vi "Render List.vi"(10 "Value":i32, 11 "Display State In":T2={"Persistent"={"Elements"=[], "PicElements"=[], "Limits"=[], "Selection"=[], "Selection Color"=0, "Highlight"=[], "Highlight Val"=0, "Highlight Color"={"Back"=0, "Edge"=0}, "Font"={"Details"={"Font Name:"="Lucida Sans", "Size"=24, "Strikeout?"=FALSE, "Italic?"=FALSE, "Underline?"=FALSE, "Outline?"=FALSE, "Shadow?"=FALSE, "Bold?"=TRUE}, "Color"=7697781}, "Bakground Color"=0}, "List Ref"=refnum, "nbVisible"=0, "FirstIdx"=0, "More.Width"=0} caption="State") -> (0 "OutOfBounds":bool, 2 "Selection":picture, 3 "Display State Out":T2={"Persistent"={"Elements"=[], "PicElements"=[], "Limits"=[], "Selection"=[], "Selection Color"=0, "Highlight"=[], "Highlight Val"=0, "Highlight Color"={"Back"=0, "Edge"=0}, "Font"={"Details"={"Font Name:"="Lucida Sans", "Size"=24, "Strikeout?"=FALSE, "Italic?"=FALSE, "Underline?"=FALSE, "Outline?"=FALSE, "Shadow?"=FALSE, "Bold?"=TRUE}, "Color"=7697781}, "Bakground Color"=0}, "List Ref"=refnum, "nbVisible"=0, "FirstIdx"=0, "More.Width"=0} caption="State", 5 "Actual Value":T1 caption="s? t:f")   [LabVIEW 2016, in "Horizontal MenuList.xctl"]
uses:
  Horizontal MenuList.xctl
  Horizontal MenuList_State.ctl
  Highlight Colors.ctl
  Horizontal MenuList_Data.ctl
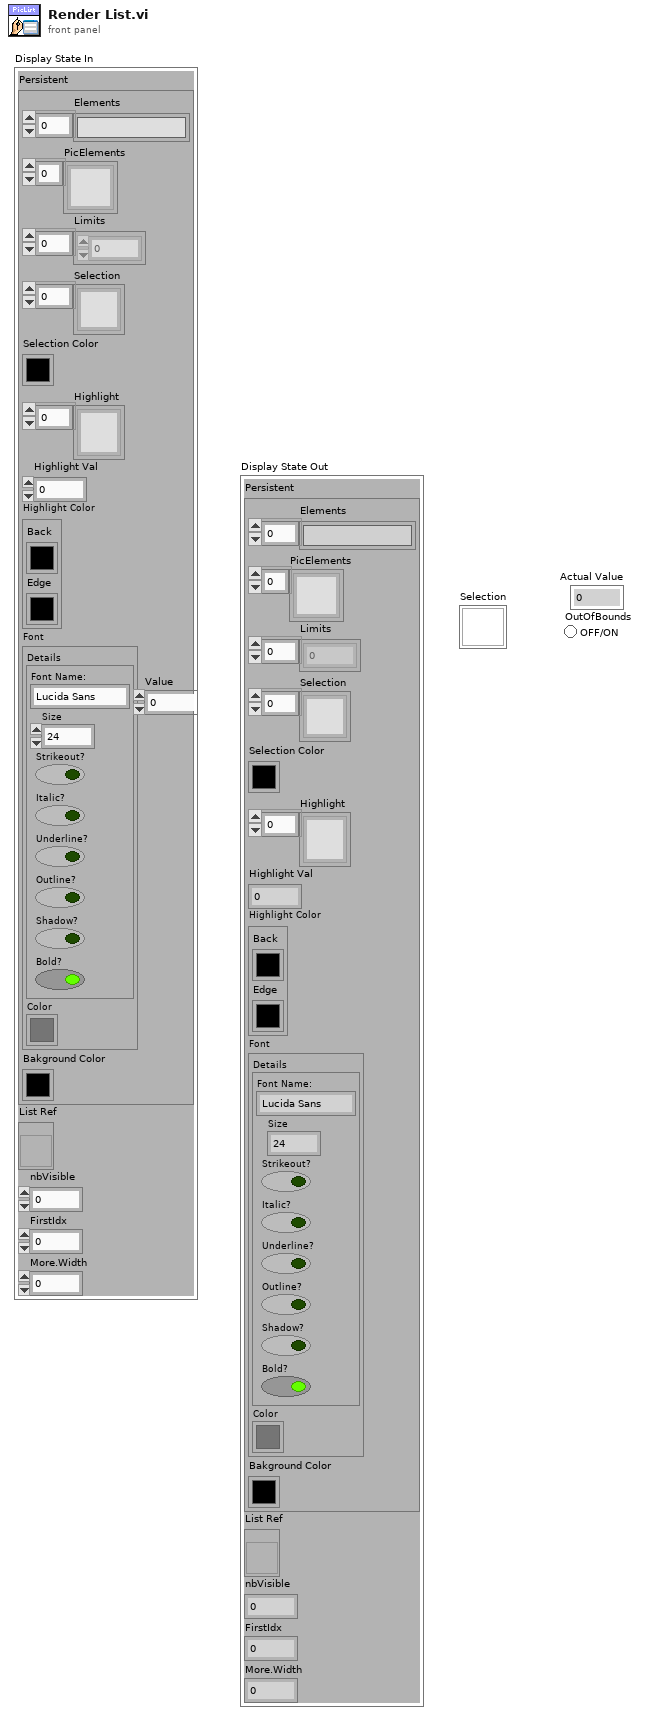
[diagram p1: front panel]
types:
  T1 = typedef "Horizontal MenuList.xctl/Horizontal MenuList_Data.ctl" = i32
  T2 = typedef "Horizontal MenuList.xctl/Horizontal MenuList_State.ctl" = cluster{"Persistent":cluster{"Elements":string[], "PicElements":picture[], "Limits":i32[], "Selection":picture[], "Selection Color":u32, "Highlight":picture[], "Highlight Val":i32, "Highlight Color":T3, "Font":cluster{"Details":cluster{"Font Name:":string, "Size":i16, "Strikeout?":bool, "Italic?":bool, "Underline?":bool, "Outline?":bool, "Shadow?":bool, "Bold?":bool}, "Color":u32}, "Bakground Color":u32}, "List Ref":refnum<vi>, "nbVisible":u8, "FirstIdx":u8, "More.Width":u8}
  T3 = typedef "Horizontal MenuList.xctl/Highlight Colors.ctl" = cluster{"Back":u32, "Edge":u32}
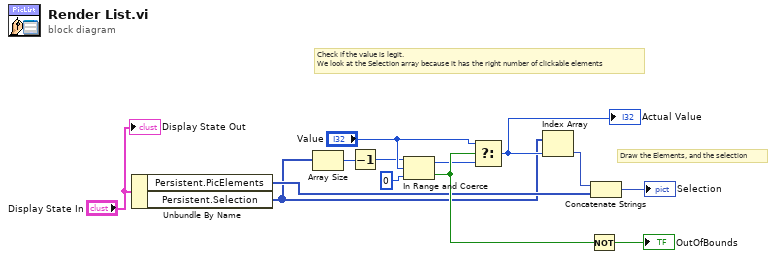
[diagram p0: block diagram]
diagram:
  # "Draw the Elements, and the selection"
  # "Check if the value is legit.\nWe look at the Selection array because it has the right number of clickable elements"
  n1 = Unbundle By Name("Display State In") -> ("Persistent.PicElements"=w4:picture[], "Persistent.Selection"=w3:picture[])
  n2 = Array Size(array=w3) -> (size(s)=w10:i32)
  n3 = Decrement(x=w10) -> (x-1=w2:i32)
  n4 = In Range and Coerce(upper limit=w2, x="Value", lower limit=T1 0) -> (coerced(x)=w1:T1, In Range?=w7:bool)
  n5 = Select(t="Value", s=w7, f=w1) -> (s? t:f=w5:T1)
  "Actual Value" <- w5
  n6 = Index Array(array=w3, index=w5) -> (element=w13:picture)
  n7 = Not(x=w7) -> (.not. x?=→"OutOfBounds":bool)
  n8 = Concatenate Strings(w13, w4) -> (→"Selection":picture)
  "Display State Out" <- "Display State In"
